vi "TransducerInfo.vi"(0 "refnum":refnum<file>, 11 "offset":i32) -> (2 "Tranducer Info":T1 {"bandwidth" format="%.2f"; "center freq" format="%.2f"; "start freq" format="%.2f"}, 4 "dup refnum":refnum<file>, 6 "bandwidth":sgl format="%.2e", 8 "center freq":sgl format="%.2f", 10 "start freq":sgl format="%.2f", 15 "ID":i32)   [LabVIEW 2022 SP3]
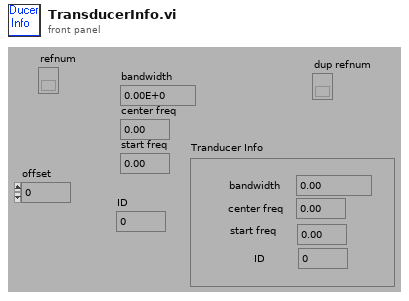
[diagram p1: front panel]
types:
  T1 = cluster{"bandwidth":sgl, "center freq":sgl, "start freq":sgl, "ID":i32}
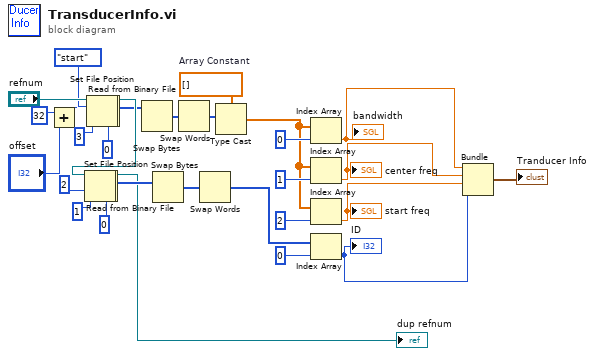
[diagram p0: block diagram]
diagram:
  w19 = sgl[] []  # Array Constant
  n1 = Add(x=32 ("pos offset (0)"), y="offset") -> (x+y=w7:i32)
  n2 = Set File Position(offset (in bytes) (0)=w7, refnum="refnum", from (0:start)=enum16{"start", "end", "current"}."start" ("pos mode (0:2)")) -> (refnum out=w2:refnum<file>, error out=w1:errorcluster)  [unwired: 1 in]
  n3 = Read from Binary File(5:0 ("byte stream type"), 8:w1, 10:3 ("count"), 11:w2) -> (2:w21:i32[], 3:w24:refnum<file>)  [unwired: 4 out]
  n4 = Set File Position(refnum=w24, from (0:start)=2) -> (refnum out=w4:refnum<file>, error out=w3:errorcluster)  [unwired: 1 in, 1 out]
  n5 = Read from Binary File(5:0 ("byte stream type"), 8:w3, 10:1 ("count"), 11:w4) -> (2:w17:i32[], 3:→"dup refnum":refnum<file>)  [unwired: 4 out]
  n6 = Swap Bytes(anything=w21) -> (byte swapped=w22:i32[])
  n7 = Swap Bytes(anything=w17) -> (byte swapped=w16:i32[])
  n8 = Swap Words(1:w22) -> (0:w18:i32[])
  n9 = Swap Words(1:w16) -> (0:w15:i32[])
  n10 = Type Cast(type=w19, x=w18) -> (*(type *) &x=w20:sgl[])
  n11 = Index Array(array=w20, index=0) -> (element=w9:sgl)
  "bandwidth" <- w9
  n12 = Index Array(array=w20, index=1) -> (element=w10:sgl)
  "center freq" <- w10
  n13 = Index Array(array=w20, index=2) -> (element=w11:sgl)
  "start freq" <- w11
  n14 = Index Array(array=w15, index=0) -> (element=w12:i32)
  "ID" <- w12
  n15 = Bundle(w9, w10, w11, "byte stream type"=w12) -> (→"Tranducer Info":cluster{sgl, sgl, sgl, "byte stream type":i32})  [unwired: 1 out]
